vi "anCntrlRefs.vi"(11 "CntrlRefs":T1) -> (3 "CntrlRefs":T1)   [LabVIEW 2014]
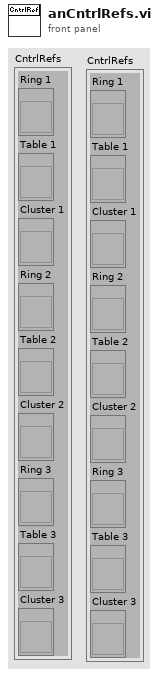
[diagram p1: front panel]
types:
  T1 = cluster{"Ring 1":refnum<vi>, "Table 1":refnum<vi>, "Cluster 1":refnum<vi>, "Ring 2":refnum<vi>, "Table 2":refnum<vi>, "Cluster 2":refnum<vi>, "Ring 3":refnum<vi>, "Table 3":refnum<vi>, "Cluster 3":refnum<vi>}
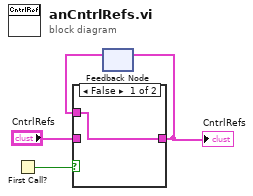
[diagram p0: block diagram]
diagram:
  n1 = First Call?() -> (First Call?: T/F=w4:bool)
  n2 = feedback #1() -> (w1:T1)  [unwired: 1 in]
  n3 = case shown="False" w4 {
    tunnel: "CntrlRefs" -> [_ w6]
    tunnel: [w5 w6] -> w2
    tunnel: w1 -> [w5 _]
    frame False {
    }
    frame True {
    }
  }
  "CntrlRefs" <- w2
  n4 = feedback-in #1(w2) -> ()
